vi "Centauro LED Low Level Parser.vi"(8 "error in (no error)":errorcluster, 9 "Read ERD List":T3[](array[typedef])=[{"ERD Number"=61758, "Data Type"=enum."string"}, {"ERD Number"=61755, "Data Type"=enum."string"}, {"ERD Number"=61757, "Data Type"=enum."string"}, {"ERD Number"=61756, "Data Type"=enum."string"}, {"ERD Number"=61751, "Data Type"=enum."string"}] {"ERD Number" format="%.0x"}, 10 "Raw Data In":string) -> (0 "error out":errorcluster, 1 "Binary Number":u32, 2 "LED Status":T2)   [LabVIEW 2016]
uses:
  Common/LabVIEW GEA2 Toolkit/LabVIEW_GEA2_Toolkit.lvlibp/type defs/ERD Read Data In.ctl
  Common/LabVIEW GEA2 Toolkit/LabVIEW_GEA2_Toolkit.lvlibp/type defs/Data Type.ctl
  type defs/LED Status OOB.ctl
  Common/LabVIEW GEA2 Toolkit/LabVIEW_GEA2_Toolkit.lvlibp
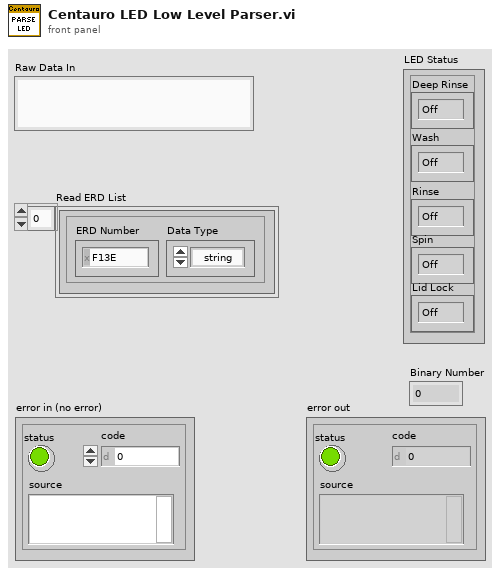
[diagram p1: front panel]
types:
  T1 = typedef "LED Status OOB.ctl" = enum32{"Off", "On", "Blink"}
  T2 = cluster{"Deep Rinse":T1, "Wash":T1, "Rinse":T1, "Spin":T1, "Lid Lock":T1}
  T3 = typedef "LabVIEW_GEA2_Toolkit.lvlibp/ERD Read Data In.ctl" = cluster{"ERD Number":u16, "Data Type":T4}
  T4 = typedef "LabVIEW_GEA2_Toolkit.lvlibp/Data Type.ctl" = enum16{"string", "boolean", "uint8_t", "uint16_t", "uint32_t", "uint64_t", "int8_t", "int16_t", "int32_t", "int64_t"}
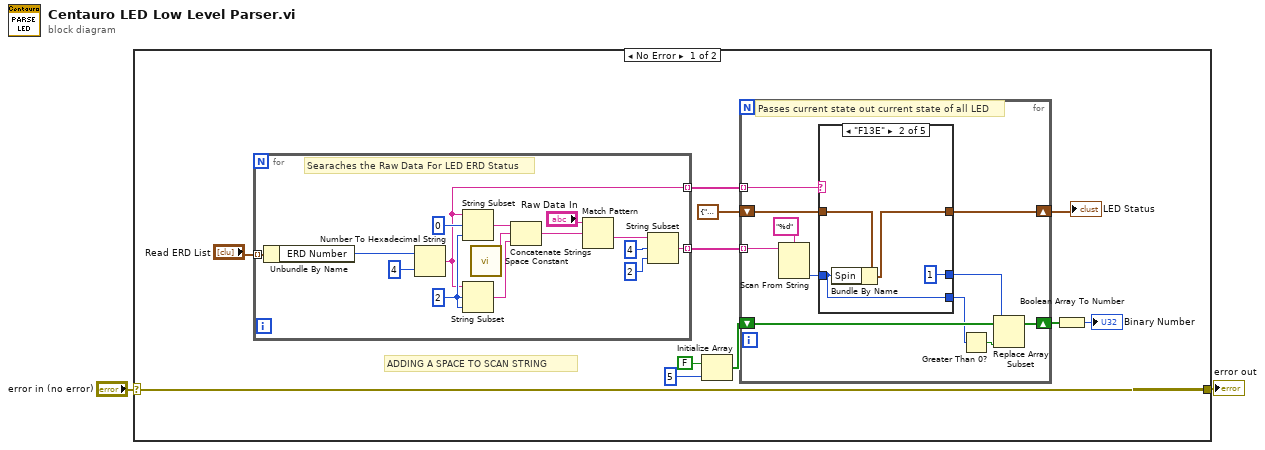
[diagram p0: block diagram]
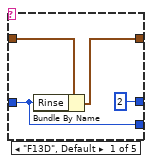
[diagram p2: hidden frame]
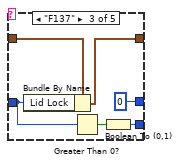
[diagram p3: hidden frame]
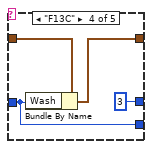
[diagram p4: hidden frame]
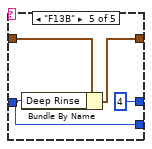
[diagram p5: hidden frame]
diagram:
  n1 = case shown="No Error" "error in (no error)" {
    selector: "error in (no error)" -> [w8 w62]
    tunnel: [w8 w62] -> w1
    frame No Error {
      # "ADDING A SPACE TO SCAN STRING"
      n2 = for {
        tunnel: "Read ERD List" -> [w28] mode=indexing
        tunnel: [w22] -> w11 mode=indexing
        tunnel: [w18] -> w10 mode=indexing
        w20 = 2 ("offset (0)")
        # "Searaches the Raw Data For LED ERD Status"
        n3 = Unbundle By Name(w28) -> ("ERD Number"=w26:u16)
        n4 = Number To Hexadecimal String(1:i16 4 ("width (-)"), 2:w26) -> (0:w18:string)
        n5 = String Subset(string=w18, offset (0)=0 ("length (rest)"), length (rest)=w20) -> (substring=w17:string)
        n6 = String Subset(string=w18, offset (0)=w20, length (rest)=w20) -> (substring=w21:string)
        n7 = call <vilib>:"Space Constant.vi"() -> ("String"=w16:string)
        n8 = Concatenate Strings(w17, w16, w21) -> (w15:string)
        n9 = Match Pattern(string="Raw Data In", regular expression=w15) -> (after substring=w23:string)  [unwired: 1 in, 3 out]
        n10 = String Subset(string=w23, offset (0)=4 ("length (rest)"), length (rest)=2 ("offset (0)")) -> (substring=w22:string)
      }
      n11 = Initialize Array(FALSE ("x > 0?"), 5 ("dimension size")) -> (w4:bool[])
      n12 = for {
        shift-right: [w38] -> w9
        shift-left: T2 {"Deep Rinse"=enum."Off", "Wash"=enum."Off", "Rinse"=enum."Off", "Spin"=enum."Off", "Lid Lock"=enum."Off"} ("LED Status 2") -> [w39]
        tunnel: w11 -> [w36] mode=indexing
        tunnel: w10 -> [w35] mode=indexing
        shift-right: [w32] -> w3
        shift-left: w4 -> [w33]
        # "Passes current state out current state of all LED"
        n13 = Scan From String(format string="%d", input string=w36) -> (output 1=w31:i32)  [unwired: 3 in, 3 out]
        n14 = case shown="\"F13E\"" w35 {
          tunnel: w39 -> [w43 w47 w53 w57 w61]
          tunnel: [w42 w46 w52 w56 w60] -> w38
          tunnel: w31 -> [w41 w45 w48 w55 w59]
          tunnel: [w41 w45 w50 w55 w59] -> w30
          tunnel: [2 ("index") 1 ("index") 0 ("index") 3 ("index") 4 ("index")] -> w29
          frame "F13D", Default {
            n15 = Bundle By Name(cluster=w43, "Rinse"=w41) -> (w42:T2)
          }
          frame "F13E" {
            n16 = Bundle By Name(cluster=w47, "Spin"=w45) -> (w46:T2)
          }
          frame "F137" {
            n17 = Bundle By Name(cluster=w53, "Lid Lock"=w48) -> (w52:T2)
            n18 = Greater Than 0?(x=w48) -> (x > 0?=w51:bool)
            n19 = Boolean To (0,1)(Boolean=w51) -> (0, 1=w50:i16)
          }
          frame "F13C" {
            n20 = Bundle By Name(cluster=w57, "Wash"=w55) -> (w56:T2)
          }
          frame "F13B" {
            n21 = Bundle By Name(cluster=w61, "Deep Rinse"=w59) -> (w60:T2)
          }
        }
        n22 = Greater Than 0?(x=w30) -> (x > 0?=w34:bool)
        n23 = Replace Array Subset(array=w33, new element=w34, index=w29) -> (w32:bool[])
      }
      "LED Status" <- w9
      n24 = Boolean Array To Number(Boolean array=w3) -> (number=→"Binary Number":u32)
    }
    frame Error {
    }
  }
  "error out" <- w1
